vi "Periodic Tasks.vi"(8 "error in":errorcluster) -> ()   [LabVIEW 2019]
doc: "This VI runs in parallel to other tasks. It can contain as many user-defined periodic loops as you need. These can carry out PID or other sorts of timed response."
uses:
  <vilib>/Rock Robotics/WPI/DriverStation/WPI_DriverStationRobotMode2.ctl
  <vilib>/Rock Robotics/Network Tables/NT Write Number.vi
  Robot Global Data.vi
  <vilib>/Rock Robotics/Network Tables/NT Write Boolean.vi
  <vilib>/Rock Robotics/WPI/ThirdParty/REV Robotics/SPARK MAX/Typedef/Spark MAX Control Type.ctl
  <vilib>/Rock Robotics/Network Tables/NT Write Numeric Array.vi
  <vilib>/Rock Robotics/WPI/RobotDrive/WPI_RobotDriveArcadeDrive_Standard(NoSaturation).vi
  <vilib>/Rock Robotics/Network Tables/NT Read Boolean.vi
panel:
  in  "error in 2":errorcluster
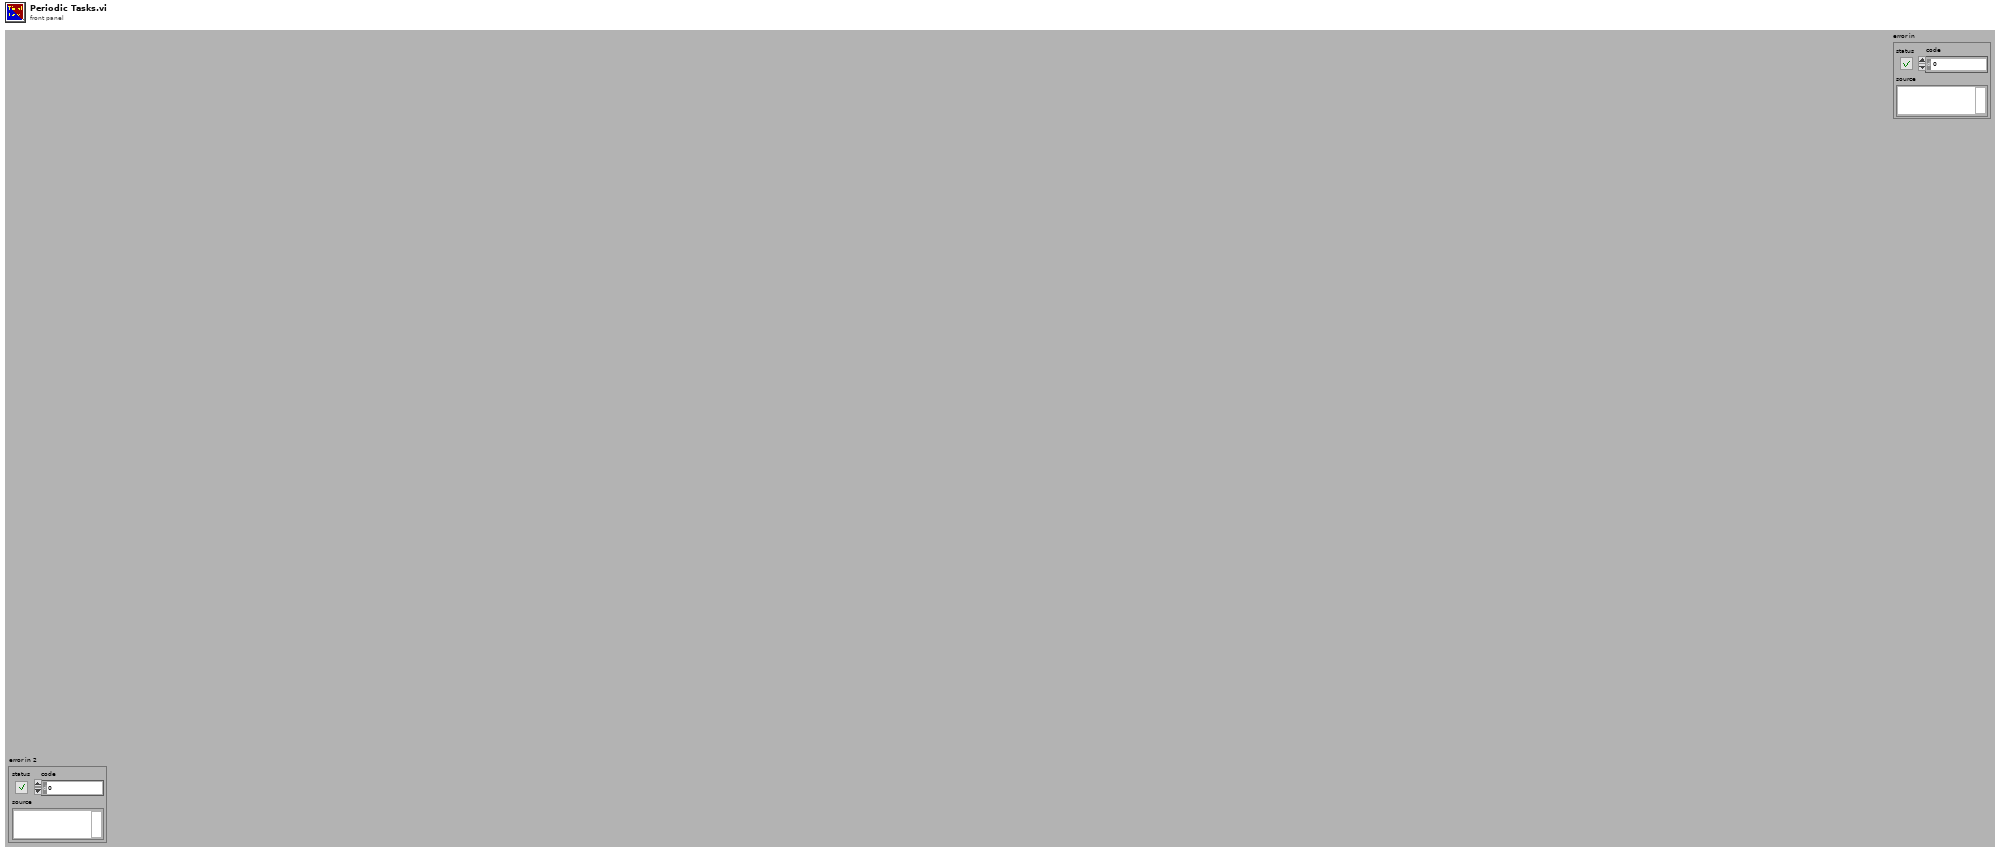
[diagram p1: front panel]
types:
  T1 = typedef "WPI_MotorControlDeviceRef.ctl" = cluster{"DeviceStatus":errorcluster, "Type":T2, "PWM":cluster{"PWM Channel":T3, "DeadBand":T4}, "CAN":cluster{"Device Number":u8, "SetOutput VI Ref":variant, "GetOutput VI Ref":variant, "Enable VI Ref":variant, "Disable VI Ref":variant, "Data":variant}, "Invert":bool, "DIO PWM":cluster{"PWM \"Enable\" Channel":T3, "DIOChannel":T5, "PWM Rate":dbl}}
  T2 = typedef "WPI_MotorControlType.ctl" = enum16{"PWM", "CAN", "DIO PWM"}
  T3 = typedef "FPGA_DIOPWMChannel.ctl" = enum8{"PWM 0", "PWM 1", "PWM 2", "PWM 3", "PWM 4", "PWM 5", "PWM 6", "PWM 7", "PWM 8", "PWM 9", "PWM MXP 0", "PWM MXP 1", "PWM MXP 2", "PWM MXP 3", "PWM MXP 4", "PWM MXP 5", "PWM MXP 6", "PWM MXP 7", "PWM MXP 8", "PWM MXP 9", "Invalid"}
  T4 = typedef "WPI_PWMDeadband.ctl" = cluster{"Name":string, "maxPositivePwm":i32, "minPositivePwm":i32, "centerPwm":i32, "maxNegativePwm":i32, "minNegativePwm":i32, "angularRange":u16}
  T5 = typedef "FPGA_DIOChannel.ctl" = enum8{"DIO 0", "DIO 1", "DIO 2", "DIO 3", "DIO 4", "DIO 5", "DIO 6", "DIO 7", "DIO 8", "DIO 9", "DIO MXP 0", "DIO MXP 1", "DIO MXP 2", "DIO MXP 3", "DIO MXP 4", "DIO MXP 5", "DIO MXP 6", "DIO MXP 7", "DIO MXP 8", "DIO MXP 9", "DIO MXP 10", "DIO MXP 11", "DIO MXP 12", "DIO MXP 13", "DIO MXP 14", "DIO MXP 15", "SPI Port CS1", "SPI Port CS2", "SPI Port CS3", "SPI Port MISO", "SPI Port MOSI", "Invalid"}
  T6 = typedef "WPI_RobotDriveDevRef.ctl" = cluster{"DevStatus":errorcluster, "Motors[]":T1[], "Square Inputs":bool, "Max Output":dbl}
  T7 = typedef "WPI_JoystickDevRef.ctl" = cluster{"Device":T8}
  T8 = typedef "WPI_JoystickDeviceEnum.ctl" = enum16{"USB 0", "USB 1", "USB 2", "USB 3", "USB 4", "USB 5"}
  T9 = typedef "WPI_ServoDeviceRef.ctl" = cluster{"DeviceStatus":errorcluster, "PWM Channel":T3, "DeadBand":T4}
  T10 = typedef "WPI_DriverStationRobotMode2.ctl" = enum16{"Autonomous Disabled", "Autonomous Enabled", "Teleop Disabled", "Teleop Enabled", "Disconnected", "Finish", "Test Disabled", "Test Enabled", "Emergency Stopped"}
  T11 = cluster{"P Gain":dbl, "I Gain":dbl, "D Gain":dbl, "F Gain":dbl, "I Zone":dbl, "Min Output":dbl, "Max Output":dbl}
  T12 = typedef "Spark MAX Control Type.ctl" = enum16{"Percent VBus", "Voltage", "Velocity", "Position", "Smart Motion", "Current", "Smart Velocity"}
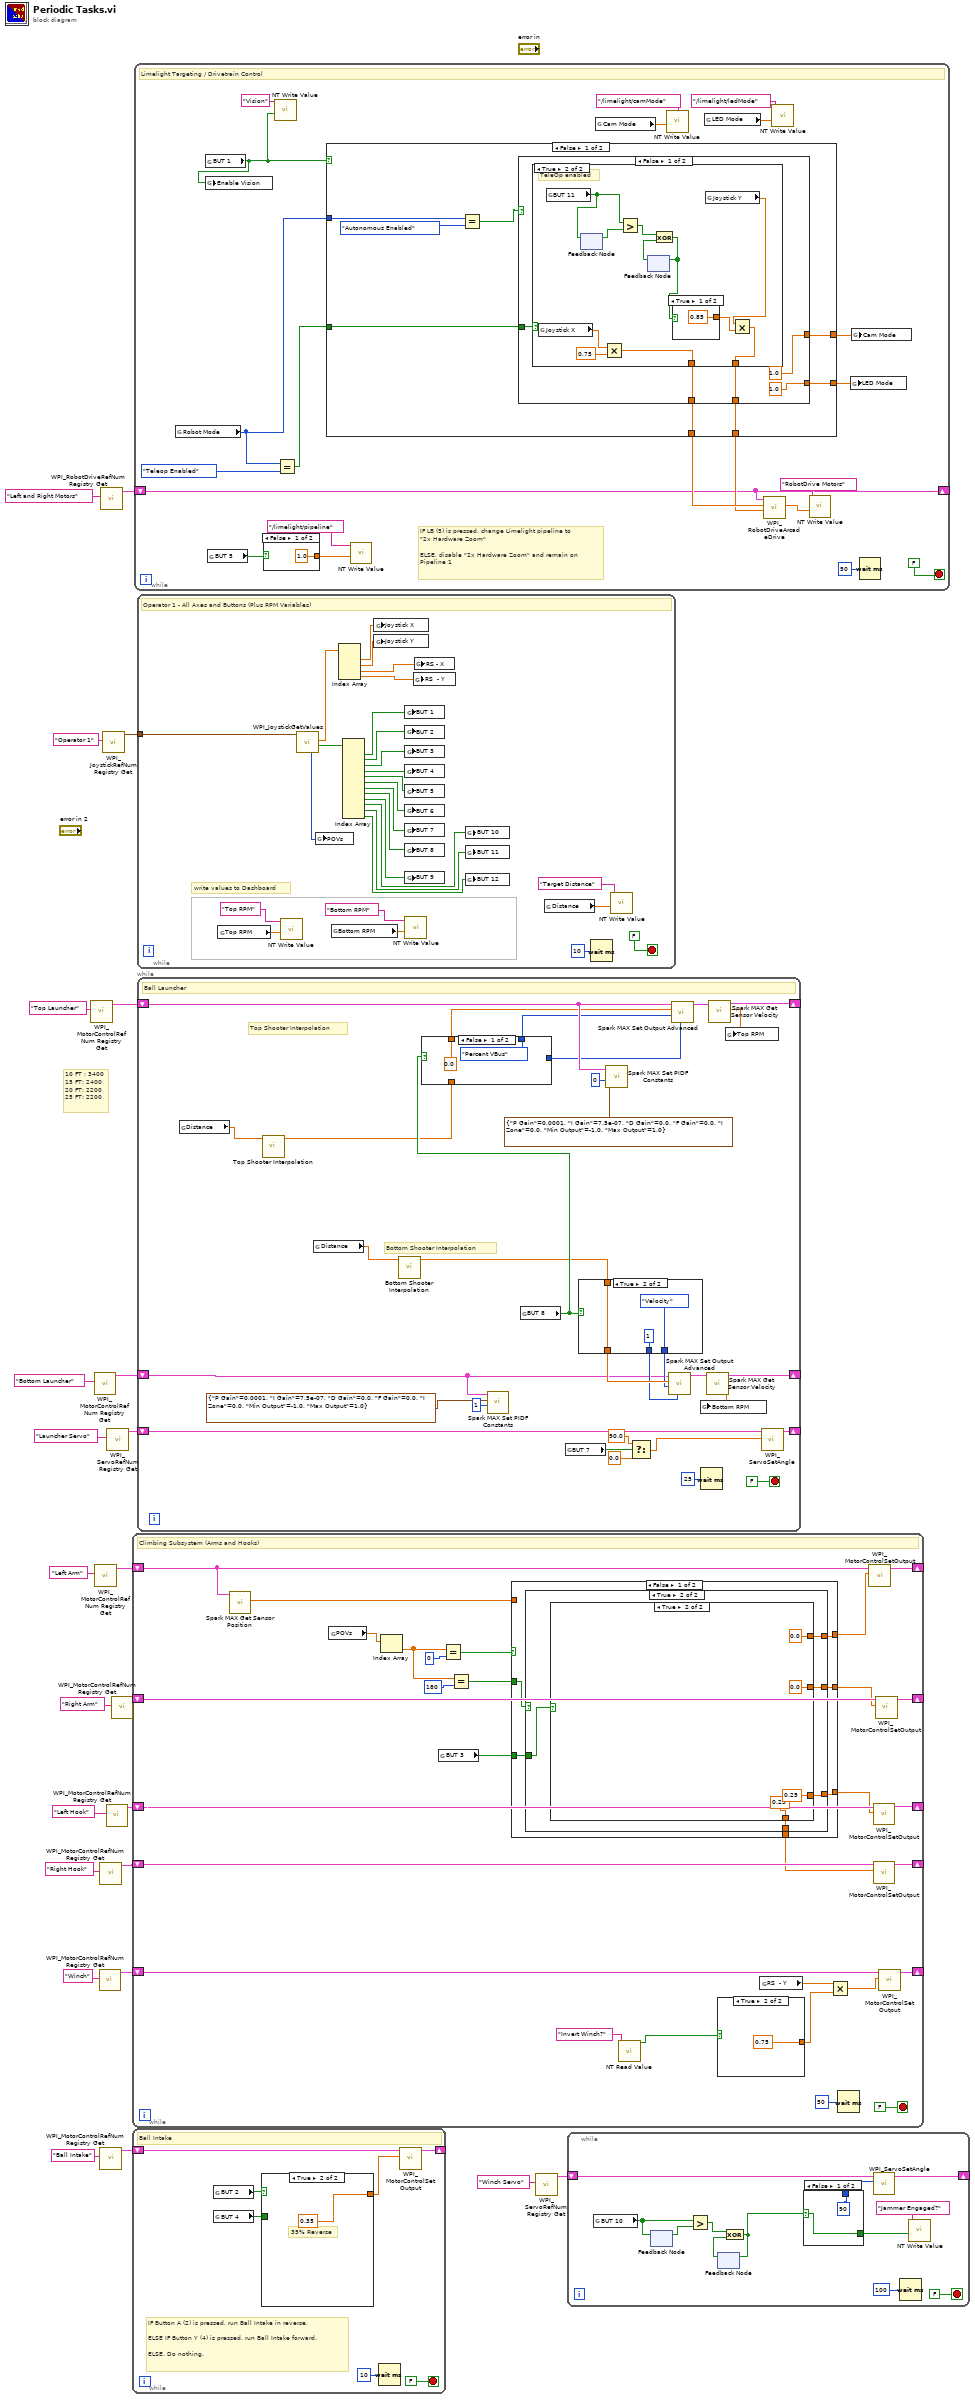
[diagram p0: block diagram]
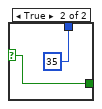
[diagram p2: hidden frame]
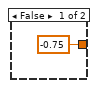
[diagram p3: hidden frame]
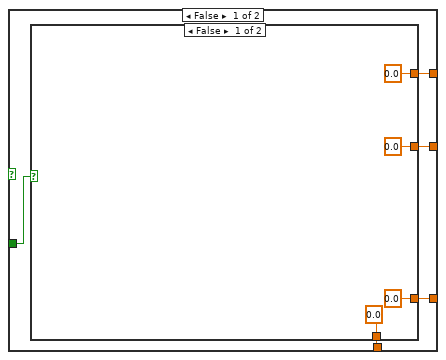
[diagram p4: hidden frame]
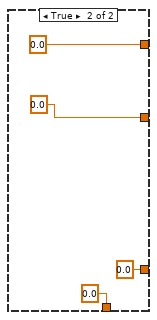
[diagram p5: hidden frame]
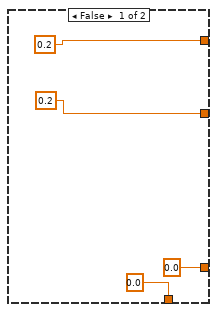
[diagram p6: hidden frame]
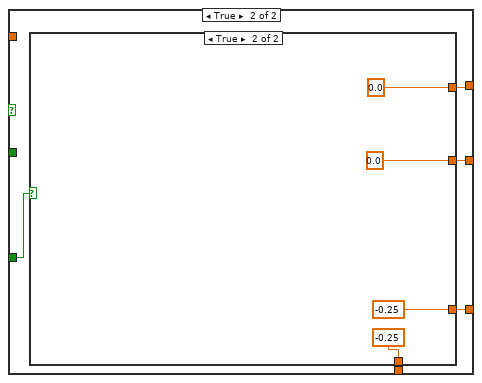
[diagram p7: hidden frame]
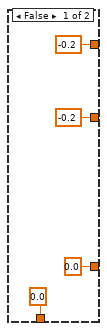
[diagram p8: hidden frame]
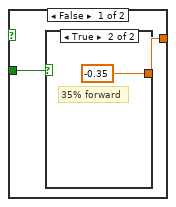
[diagram p9: hidden frame]
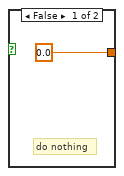
[diagram p10: hidden frame]
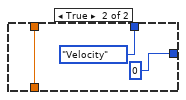
[diagram p11: hidden frame]
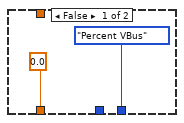
[diagram p12: hidden frame]
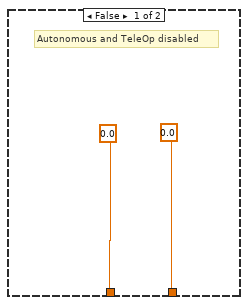
[diagram p13: hidden frame]
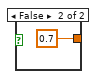
[diagram p14: hidden frame]
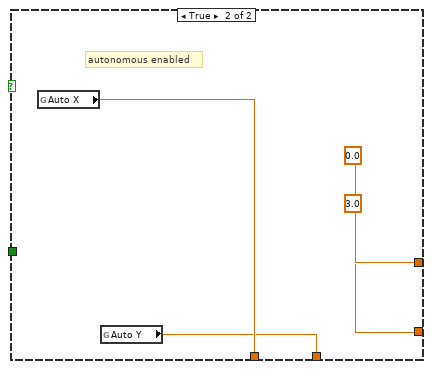
[diagram p15: hidden frame]
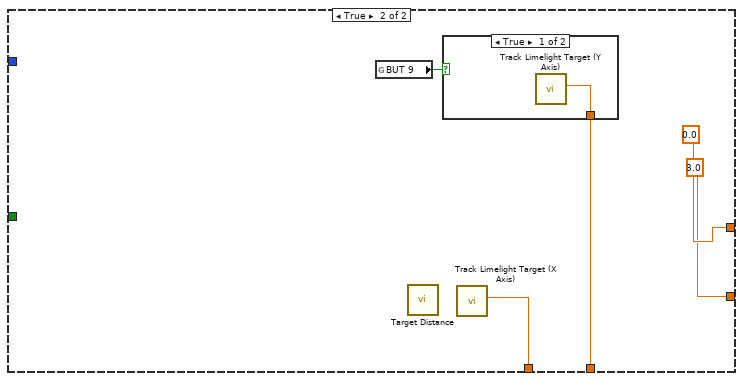
[diagram p16: hidden frame]
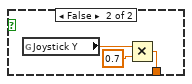
[diagram p17: hidden frame]
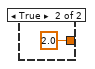
[diagram p18: hidden frame]
diagram:
  # "10 FT : 3400\n15 FT: 2400\n20 FT: 2200\n25 FT: 2200"
  n1 = call <vilib>:"WPI_MotorControlRefNum Registry Get.vi"("refnum name"="Top Launcher") -> ("MotorControlDevRef"=w19:T1)  [unwired: 9 in, 1 out]
  n2 = call <vilib>:"WPI_MotorControlRefNum Registry Get.vi"("refnum name"="Bottom Launcher") -> ("MotorControlDevRef"=w21:T1)  [unwired: 9 in, 1 out]
  n3 = call <vilib>:"WPI_MotorControlRefNum Registry Get.vi"("refnum name"="Left Arm") -> ("MotorControlDevRef"=w13:T1)  [unwired: 9 in, 1 out]
  n4 = call <vilib>:"WPI_MotorControlRefNum Registry Get.vi"("refnum name"="Winch") -> ("MotorControlDevRef"=w5:T1)  [unwired: 9 in, 1 out]
  n5 = call <vilib>:"WPI_MotorControlRefNum Registry Get.vi"("refnum name"="Right Hook") -> ("MotorControlDevRef"=w10:T1)  [unwired: 9 in, 1 out]
  n6 = call <vilib>:"WPI_MotorControlRefNum Registry Get.vi"("refnum name"="Ball Intake") -> ("MotorControlDevRef"=w15:T1)  [unwired: 9 in, 1 out]
  n7 = call <vilib>:"WPI_RobotDriveRefNum Registry Get.vi"("refnum name"="Left and Right Motors") -> ("RobotDriveDevRef"=w23:T6)  [unwired: 1 in, 9 out]
  n8 = call <vilib>:"WPI_JoystickRefNum Registry Get.vi"("refnum name"="Operator 1") -> ("JoystickDevRef"=w1:T7)  [unwired: 1 in, 9 out]
  n9 = call <vilib>:"WPI_MotorControlRefNum Registry Get.vi"("refnum name"="Left Hook") -> ("MotorControlDevRef"=w11:T1)  [unwired: 9 in, 1 out]
  n10 = call <vilib>:"WPI_ServoRefNum Registry Get.vi"("refnum name"="Launcher Servo") -> ("ServoDeviceRef"=w17:T9)  [unwired: 9 in, 1 out]
  n11 = call <vilib>:"WPI_MotorControlRefNum Registry Get.vi"("refnum name"="Right Arm") -> ("MotorControlDevRef"=w12:T1)  [unwired: 9 in, 1 out]
  n12 = while {
    shift-right: [w46] -> _
    shift-left: w13 -> [w31]
    shift-right: [w47] -> _
    shift-left: w12 -> [w32]
    shift-right: [w50] -> _
    shift-left: w10 -> [w49]
    shift-right: [w51] -> _
    shift-left: w11 -> [w48]
    shift-right: [w37] -> _
    shift-left: w5 -> [w36]
    stop <- FALSE stop-if-true
    # "Climbing Subsystem (Arms and Hooks)"
    n13 = call <vilib>:"Spark MAX Get Sensor Position.vi"("MotorControlDevRef in"=w31) -> ("Sensor Position"=w45:dbl)  [unwired: 7 in, 3 out]
    n14 = global read "Robot Global Data.vi" "POVs"() -> (w44:dbl[])
    n15 = Index Array(array=w44) -> (element=w38:dbl)  [unwired: 1 in]
    n16 = global read "Robot Global Data.vi" "BUT 3"() -> (w39:bool)
    n17 = Equal?(x=w38, y=i16 0) -> (x = y?=w41:bool)
    n18 = Equal?(x=w38, y=i16 180) -> (x = y?=w40:bool)
    n19 = case shown="False" w41 {
      tunnel: w40 -> [w61 _]
      tunnel: w39 -> [w60 w88]
      tunnel: w45 -> [_ _]
      tunnel: [w59 w92] -> w30
      tunnel: [w58 w91] -> w29
      tunnel: [w57 w90] -> w28
      tunnel: [w56 w89] -> w27
      frame False {
        n20 = case shown="True" w61 {
          tunnel: w60 -> [w62 w79]
          tunnel: [w66 w78] -> w59
          tunnel: [w65 w77] -> w58
          tunnel: [w64 w76] -> w57
          tunnel: [w63 w75] -> w56
          frame False {
            n21 = case shown="False" w62 {
              tunnel: [0.0 ("Output") 0.0 ("Output")] -> w66
              tunnel: [0.0 ("Output") 0.0 ("Output")] -> w65
              tunnel: [0.0 ("Output") 0.0 ("Output")] -> w64
              tunnel: [0.0 ("Output") 0.0 ("Output")] -> w63
              frame False {
              }
              frame True {
              }
            }
          }
          frame True {
            n22 = case shown="True" w79 {
              tunnel: [0.2 ("Output") 0.0 ("Output")] -> w78
              tunnel: [0.2 ("Output") 0.0 ("Output")] -> w77
              tunnel: [0.0 ("Output") 0.25 ("Output")] -> w76
              tunnel: [0.0 ("Output") 0.25 ("Output")] -> w75
              frame False {
              }
              frame True {
              }
            }
          }
        }
      }
      frame True {
        n23 = case shown="True" w88 {
          tunnel: [-0.2 ("Output") 0.0 ("Output")] -> w92
          tunnel: [-0.2 ("Output") 0.0 ("Output")] -> w91
          tunnel: [0.0 ("Output") -0.25 ("Output")] -> w90
          tunnel: [0.0 ("Output") -0.25 ("Output")] -> w89
          frame False {
          }
          frame True {
          }
        }
      }
    }
    n24 = call-poly <vilib>:"NT Read Value.vi"("Name"="Invert Winch?") -> ("Boolean"=w25:bool)  [unwired: 9 in, 1 out]
    n25 = case shown="True" w25 {
      tunnel: [-0.75 ("y") 0.75 ("y")] -> w33
      frame False {
      }
      frame True {
      }
    }
    n26 = global read "Robot Global Data.vi" "RS  - Y"() -> (w35:dbl)
    n27 = Multiply(x=w35, y=w33) -> (x*y=w34:dbl)
    n28 = Wait (ms)(milliseconds to wait=u32 50) -> ()  [unwired: 1 out]
    n29 = call <vilib>:"WPI_MotorControlSetOutput.vi"("Output"=w30, "MotorControlDevRef"=w31) -> ("MotorControlDevRef"=w46:T1)  [unwired: 7 in, 2 out]
    n30 = call <vilib>:"WPI_MotorControlSetOutput.vi"("Output"=w28, "MotorControlDevRef"=w48) -> ("MotorControlDevRef"=w51:T1)  [unwired: 7 in, 2 out]
    n31 = call <vilib>:"WPI_MotorControlSetOutput.vi"("Output"=w27, "MotorControlDevRef"=w49) -> ("MotorControlDevRef"=w50:T1)  [unwired: 7 in, 2 out]
    n32 = call <vilib>:"WPI_MotorControlSetOutput.vi"("Output"=w29, "MotorControlDevRef"=w32) -> ("MotorControlDevRef"=w47:T1)  [unwired: 7 in, 2 out]
    n33 = call <vilib>:"WPI_MotorControlSetOutput.vi"("Output"=w34, "MotorControlDevRef"=w36) -> ("MotorControlDevRef"=w37:T1)  [unwired: 7 in, 2 out]
  }
  n34 = while {
    shift-right: [w104] -> _
    shift-left: w15 -> [w105]
    stop <- FALSE stop-if-true
    # "IF Button A (2) is pressed, run Ball Intake in reverse. \n\nELSE IF Button Y (4) is pressed, run Ball Intake forward.\n\nELSE, Do nothing."
    # "Ball Intake"
    n35 = global read "Robot Global Data.vi" "BUT 2"() -> (w102:bool)
    n36 = global read "Robot Global Data.vi" "BUT 4"() -> (w103:bool)
    n37 = case shown="True" w102 {
      tunnel: [w109 0.35 ("Output")] -> w101
      tunnel: w103 -> [w108 _]
      frame False {
        n38 = case shown="True" w108 {
          tunnel: [0.0 ("Output") -0.35 ("Output")] -> w109
          frame False {
            # "do nothing"
          }
          frame True {
            # "35% forward"
          }
        }
      }
      frame True {
        # "35% Reverse"
      }
    }
    n39 = Wait (ms)(milliseconds to wait=u32 10) -> ()  [unwired: 1 out]
    n40 = call <vilib>:"WPI_MotorControlSetOutput.vi"("Output"=w101, "MotorControlDevRef"=w105) -> ("MotorControlDevRef"=w104:T1)  [unwired: 7 in, 2 out]
  }
  n41 = while {
    shift-right: [w124] -> _
    shift-left: w23 -> [w124]
    stop <- FALSE stop-if-true
    # "IF LB (5) is pressed, change Limelight pipeline to \n\"2x Hardware Zoom\"\n\nELSE, disable \"2x Hardware Zoom\" and remain on\nPipeline 1"
    # "Limelight Targeting / Drivetrain Control"
    n42 = global read "Robot Global Data.vi" "Robot Mode"() -> (w114:T10)
    n43 = global read "Robot Global Data.vi" "BUT 1"() -> (w122:bool)
    n44 = global write "Robot Global Data.vi" "Enable Vision"(w122) -> ()
    n45 = global read "Robot Global Data.vi" "BUT 5"() -> (w127:bool)
    n46 = case shown="False" w127 {
      tunnel: [1.0 ("Numeric") 2.0 ("Numeric")] -> w130
      frame False {
      }
      frame True {
      }
    }
    n47 = call-poly <vilib>:"NT Write Value.vi"("Boolean"=w122, "Name"="Vision") -> ()  [unwired: 9 in, 1 out]
    n48 = Equal?(x=w114, y=WPI_DriverStationRobotMode2."Teleop Enabled") -> (x = y?=w115:bool)
    n49 = case shown="False" w122 {
      tunnel: [w141 w170] -> w128
      tunnel: [w140 w169] -> w129
      tunnel: [w139 0.0 ("Numeric")] -> w117
      tunnel: [w138 3.0 ("Numeric")] -> w116
      tunnel: w115 -> [w136 _]
      tunnel: w114 -> [w135 _]
      frame False {
        n50 = Equal?(x=w135, y=WPI_DriverStationRobotMode2."Autonomous Enabled") -> (x = y?=w137:bool)
        n51 = case shown="False" w137 {
          tunnel: [w145 w162] -> w141
          tunnel: [w146 w163] -> w140
          tunnel: [1.0 ("Numeric") 0.0 ("Numeric")] -> w139
          tunnel: [1.0 ("Numeric") 3.0 ("Numeric")] -> w138
          tunnel: w136 -> [w142 _]
          frame False {
            n52 = case shown="True" w142 {
              tunnel: [0.0 ("Joystick X") w157] -> w146
              tunnel: [0.0 ("Joystick Y") w155] -> w145
              frame False {
                # "Autonomous and TeleOp disabled"
              }
              frame True {
                # "TeleOp enabled"
                n53 = global read "Robot Global Data.vi" "Joystick X"() -> (w159:dbl)
                n54 = global read "Robot Global Data.vi" "BUT 11"() -> (w151:bool)
                n55 = feedback #1() -> (w150:bool)  [unwired: 1 in]
                n56 = feedback-in #1(w151) -> ()
                n57 = Multiply(x=w159, y=0.75) -> (x*y=w157:dbl)
                n58 = Greater?(x=w151, y=w150) -> (0:w153:bool)
                n59 = feedback #2() -> (w152:bool)  [unwired: 1 in]
                n60 = Exclusive Or(1:w152, 2:w153) -> (0:w149:bool)
                n61 = feedback-in #2(w149) -> ()
                n62 = case shown="True" w149 {
                  tunnel: [0.85 ("y") 0.7 ("y")] -> w154
                  frame True {
                  }
                  frame False {
                  }
                }
                n63 = global read "Robot Global Data.vi" "Joystick Y"() -> (w156:dbl)
                n64 = Multiply(x=w156, y=w154) -> (x*y=w155:dbl)
              }
            }
          }
          frame True {
            # "autonomous enabled"
            n65 = global read "Robot Global Data.vi" "Auto X"() -> (w163:dbl)
            n66 = global read "Robot Global Data.vi" "Auto Y"() -> (w162:dbl)
          }
        }
      }
      frame True {
        n67 = global read "Robot Global Data.vi" "BUT 9"() -> (w166:bool)
        n68 = call "Target Distance.vi"() -> ()  [unwired: 12 in]
        n69 = case shown="True" w166 {
          tunnel: [w171 w174] -> w170
          frame True {
            n70 = call "Track Limelight Target (Y Axis).vi"() -> ("Joystick Y"=w171:dbl)  [unwired: 11 in]
          }
          frame False {
            n71 = global read "Robot Global Data.vi" "Joystick Y"() -> (w173:dbl)
            n72 = Multiply(x=w173, y=0.7) -> (x*y=w174:dbl)
          }
        }
        n73 = call "Track Limelight Target (X Axis).vi"() -> ("Joystick X"=w169:dbl)  [unwired: 11 in]
      }
    }
    n74 = call-poly <vilib>:"NT Write Value.vi"("Numeric"=w130, "Name"="/limelight/pipeline") -> ()  [unwired: 9 in, 1 out]
    n75 = global read "Robot Global Data.vi" "Cam Mode"() -> (w120:dbl)
    n76 = call-poly <vilib>:"NT Write Value.vi"("Numeric"=w120, "Name"="/limelight/camMode" ("Camera Mode")) -> ()  [unwired: 9 in, 1 out]
    n77 = global read "Robot Global Data.vi" "LED Mode"() -> (w118:dbl)
    n78 = call-poly <vilib>:"WPI_RobotDriveArcadeDrive.vi"("Y axis value"=w128, "X axis value"=w129, "RobotDriveDevRef"=w124) -> ("Motor Values"=w125:dbl[])  [unwired: 6 in, 2 out]
    n79 = call-poly <vilib>:"NT Write Value.vi"("Numeric"=w118, "Name"="/limelight/ledMode" ("LED Mode")) -> ()  [unwired: 9 in, 1 out]
    n80 = call-poly <vilib>:"NT Write Value.vi"("Numeric Array"=w125, "Name"="RobotDrive Motors") -> ()  [unwired: 9 in, 1 out]
    n81 = global write "Robot Global Data.vi" "LED Mode"(w116) -> ()
    n82 = global write "Robot Global Data.vi" "Cam Mode"(w117) -> ()
    n83 = Wait (ms)(milliseconds to wait=u32 50) -> ()  [unwired: 1 out]
  }
  n84 = while {
    tunnel: w1 -> [w181]
    stop <- FALSE stop-if-true
    # "write values to Dashboard"
    # "Operator 1 - All Axes and Buttons (Plus RPM Variables)"
    n85 = global read "Robot Global Data.vi" "Top RPM"() -> (w186:dbl)
    n86 = call-poly <vilib>:"NT Write Value.vi"("Numeric"=w186, "Name"="Top RPM") -> ()  [unwired: 9 in, 1 out]
    n87 = call <vilib>:"WPI_JoystickGetValues.vi"("JoystickDevRef"=w181) -> ("Buttons"=w203:bool[], "Axes"=w190:dbl[], "POVs"=w182:i16[])  [unwired: 6 in, 2 out]
    n88 = global write "Robot Global Data.vi" "POVs"(w182) -> ()
    n89 = global read "Robot Global Data.vi" "Bottom RPM"() -> (w184:dbl)
    n90 = Index Array(array=w190) -> (element #1=w180:dbl, element #2=w179:dbl, element #3=w183:dbl, element #4=w189:dbl)  [unwired: 4 in]
    n91 = Index Array(array=w203) -> (element #1=w202:bool, element #2=w201:bool, element #3=w200:bool, element #4=w199:bool, element #5=w198:bool, element #6=w197:bool, element #7=w196:bool, element #8=w195:bool, element #9=w194:bool, element #10=w193:bool, element #11=w192:bool, element #12=w191:bool)  [unwired: 12 in]
    n92 = global write "Robot Global Data.vi" "Joystick X"(w180) -> ()
    n93 = global write "Robot Global Data.vi" "Joystick Y"(w179) -> ()
    n94 = global write "Robot Global Data.vi" "BUT 1"(w202) -> ()
    n95 = global write "Robot Global Data.vi" "BUT 2"(w201) -> ()
    n96 = global write "Robot Global Data.vi" "BUT 3"(w200) -> ()
    n97 = global write "Robot Global Data.vi" "BUT 4"(w199) -> ()
    n98 = global write "Robot Global Data.vi" "BUT 5"(w198) -> ()
    n99 = global write "Robot Global Data.vi" "BUT 6"(w197) -> ()
    n100 = global write "Robot Global Data.vi" "BUT 7"(w196) -> ()
    n101 = global write "Robot Global Data.vi" "BUT 8"(w195) -> ()
    n102 = global write "Robot Global Data.vi" "BUT 9"(w194) -> ()
    n103 = call-poly <vilib>:"NT Write Value.vi"("Numeric"=w184, "Name"="Bottom RPM") -> ()  [unwired: 9 in, 1 out]
    n104 = global write "Robot Global Data.vi" "RS  - Y"(w189) -> ()
    n105 = global write "Robot Global Data.vi" "RS - X"(w183) -> ()
    n106 = global write "Robot Global Data.vi" "BUT 10"(w193) -> ()
    n107 = global write "Robot Global Data.vi" "BUT 11"(w192) -> ()
    n108 = global write "Robot Global Data.vi" "BUT 12"(w191) -> ()
    n109 = global read "Robot Global Data.vi" "Distance"() -> (w178:dbl)
    n110 = Wait (ms)(milliseconds to wait=u32 10) -> ()  [unwired: 1 out]
    n111 = call-poly <vilib>:"NT Write Value.vi"("Numeric"=w178, "Name"="Target Distance") -> ()  [unwired: 9 in, 1 out]
  }
  n112 = while {
    shift-right: [w233] -> _
    shift-left: w21 -> [w210]
    shift-right: [w232] -> _
    shift-left: w19 -> [w225]
    shift-right: [w231] -> _
    shift-left: w17 -> [w226]
    stop <- FALSE stop-if-true
    # "Bottom Shooter Interpolation"
    # "Top Shooter Interpolation"
    # "Ball Launcher"
    n113 = global read "Robot Global Data.vi" "Distance"() -> (w206:dbl)
    n114 = call "Top Shooter Interpolation.vi"("Distance"=w206) -> ("interpolation value"=w215:dbl)  [unwired: 10 in]
    n115 = global read "Robot Global Data.vi" "Distance"() -> (w205:dbl)
    n116 = call "Bottom Shooter Interpolation.vi"("Distance"=w205) -> ("interpolation value"=w207:dbl)  [unwired: 10 in]
    n117 = call <vilib>:"Spark MAX Set PIDF Constants.vi"("PIDF Slot"=1, "PID Constants"=T11 {"P Gain"=0.0001, "I Gain"=7.5e-07, "D Gain"=0.0, "F Gain"=0.0, "I Zone"=0.0, "Min Output"=-1.0, "Max Output"=1.0}, "MotorControlDeviceRef"=w210) -> ()  [unwired: 7 in, 2 out]
    n118 = global read "Robot Global Data.vi" "BUT 8"() -> (w217:bool)
    n119 = case shown="False" w217 {
      tunnel: [0.0 ("Setpoint") w240] -> w216
      tunnel: w215 -> [_ w240]
      tunnel: [_ 0 ("PIDF Slot (0)")] -> w212
      tunnel: [Spark_MAX_Control_Type."Percent VBus" ("Control Mode") Spark_MAX_Control_Type."Velocity" ("Control Mode")] -> w211
      frame False {
      }
      frame True {
      }
    }
    n120 = global read "Robot Global Data.vi" "BUT 7"() -> (w230:bool)
    n121 = case shown="True" w217 {
      tunnel: [0.0 ("Setpoint") w243] -> w218
      tunnel: [_ 1 ("PIDF Slot (0)")] -> w214
      tunnel: [Spark_MAX_Control_Type."Percent VBus" ("Control Mode") Spark_MAX_Control_Type."Velocity" ("Control Mode")] -> w213
      tunnel: w207 -> [_ w243]
      frame False {
      }
      frame True {
      }
    }
    n122 = call <vilib>:"Spark MAX Set PIDF Constants.vi"("PIDF Slot"=0, "PID Constants"=T11 {"P Gain"=0.0001, "I Gain"=7.5e-07, "D Gain"=0.0, "F Gain"=0.0, "I Zone"=0.0, "Min Output"=-1.0, "Max Output"=1.0}, "MotorControlDeviceRef"=w225) -> ()  [unwired: 7 in, 2 out]
    n123 = Select(t=90.0, s=w230, f=0.0) -> (s? t:f=w227:dbl)
    n124 = call <vilib>:"Spark MAX Set Output Advanced.vi"("PIDF Slot (0)"=w214, "Control Mode"=w213, "Setpoint"=w218, "MotorControlDevRef"=w210) -> ("MotorControlDevRef"=w221:T1)  [unwired: 6 in, 1 out]
    n125 = call <vilib>:"Spark MAX Set Output Advanced.vi"("PIDF Slot (0)"=w212, "Control Mode"=w211, "Setpoint"=w216, "MotorControlDevRef"=w225) -> ("MotorControlDevRef"=w224:T1)  [unwired: 6 in, 1 out]
    n126 = Wait (ms)(milliseconds to wait=u32 25) -> ()  [unwired: 1 out]
    n127 = call <vilib>:"Spark MAX Get Sensor Velocity.vi"("MotorControlDevRef in"=w221) -> ("Sensor Velocity"=w223:dbl, "MotorControlDevRef out"=w233:T1)  [unwired: 7 in, 2 out]
    n128 = global write "Robot Global Data.vi" "Bottom RPM"(w223) -> ()
    n129 = call <vilib>:"Spark MAX Get Sensor Velocity.vi"("MotorControlDevRef in"=w224) -> ("Sensor Velocity"=w222:dbl, "MotorControlDevRef out"=w232:T1)  [unwired: 7 in, 2 out]
    n130 = global write "Robot Global Data.vi" "Top RPM"(w222) -> ()
    n131 = call <vilib>:"WPI_ServoSetAngle.vi"("Angle"=w227, "ServoDeviceRef"=w226) -> ("ServoDeviceRef"=w231:T9)  [unwired: 8 in, 1 out]
  }
  n132 = call <vilib>:"WPI_ServoRefNum Registry Get.vi"("refnum name"="Winch Servo") -> ("ServoDeviceRef"=w4:T9)  [unwired: 9 in, 1 out]
  n133 = while {
    shift-right: [w255] -> _
    shift-left: w4 -> [w254]
    stop <- FALSE stop-if-true
    n134 = global read "Robot Global Data.vi" "BUT 10"() -> (w249:bool)
    n135 = feedback-in #3(w249) -> ()
    n136 = feedback #3() -> (w250:bool)  [unwired: 1 in]
    n137 = Greater?(x=w249, y=w250) -> (0:w248:bool)
    n138 = feedback #4() -> (w247:bool)  [unwired: 1 in]
    n139 = Exclusive Or(1:w247, 2:w248) -> (0:w246:bool)
    n140 = feedback-in #4(w246) -> ()
    n141 = case shown="False" w246 {
      selector: w246 -> [w258 w260]
      tunnel: [90 ("Angle") 35 ("Angle")] -> w253
      tunnel: [w258 w260] -> w251
      frame False {
      }
      frame True {
      }
    }
    n142 = call <vilib>:"WPI_ServoSetAngle.vi"("Angle"=w253, "ServoDeviceRef"=w254) -> ("ServoDeviceRef"=w255:T9)  [unwired: 8 in, 1 out]
    n143 = Wait (ms)(milliseconds to wait=u32 100) -> ()  [unwired: 1 out]
    n144 = call-poly <vilib>:"NT Write Value.vi"("Boolean"=w251, "Name"="Jammer Engaged?") -> ()  [unwired: 9 in, 1 out]
  }
